vi "path_output.vi"() -> (1 "Path output":path caption="selected path", 2 "Error out":errorcluster)   [LabVIEW 2016]
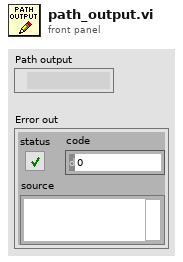
[diagram p1: front panel]
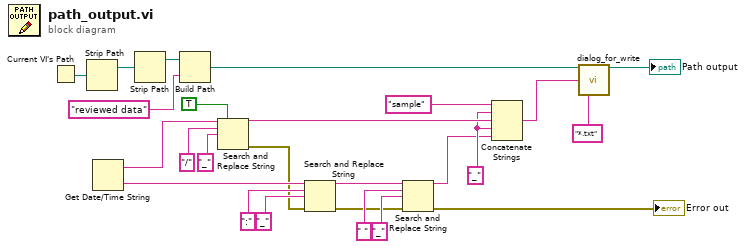
[diagram p0: block diagram]
diagram:
  w11 = "_" ("string")
  n1 = Current VI's Path() -> (path=w9:path)
  n2 = Strip Path(path=w9) -> (stripped path=w4:path)  [unwired: 1 out]
  n3 = Get Date/Time String() -> (date string=w22:string, time string=w18:string)  [unwired: 3 in]
  n4 = Strip Path(path=w4) -> (stripped path=w5:path)  [unwired: 1 out]
  n5 = Build Path(base path=w5, name or relative path="reviewed data") -> (appended path=w7:path)
  n6 = Search and Replace String(replace all?=TRUE ("replace all? (F)"), input string=w22, search string="/", replace string="_" ("replace string (\"\")")) -> (result string=w20:string, error out=w3:errorcluster)  [unwired: 4 in, 2 out]
  n7 = Search and Replace String(input string=w18, search string=":", replace string="_" ("replace string (\"\")"), error in=w3) -> (result string=w12:string, error out=w2:errorcluster)  [unwired: 4 in, 2 out]
  n8 = Search and Replace String(input string=w12, search string=" ", replace string="_" ("replace string (\"\")"), error in=w2) -> (result string=w10:string, error out=→"Error out":errorcluster)  [unwired: 4 in, 2 out]
  n9 = Concatenate Strings("sample" ("string"), w11, w20, w11, w10) -> (w23:string)
  n10 = call "dialog_for_write.vi"("start path"=w7, "default name"=w23, "pattern (all files)"="*.txt") -> ("selected path"=→"Path output":path)  [unwired: 9 in, 3 out]
